vi "Test.vi"() -> ()   [LabVIEW 2014]
panel:
  out "PLC连线成功":bool
  out "接收数据":string
  # "8000 0200 0100 00C0 0000 0101 8207 D000 0001"
  # "C0 00 02 00 C0 00 00 01 00 00 01 01 00 00 00 54"
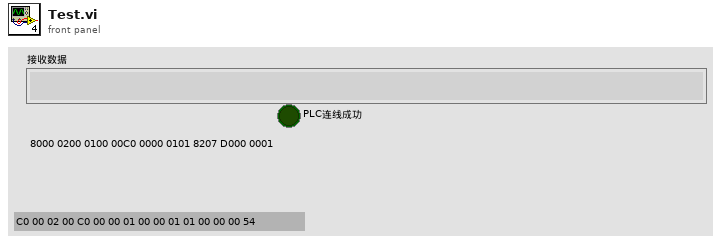
[diagram p1: front panel]
types:
  T1 = typedef "欧姆龙PLC Action.ctl" = enum16{"初始化", "重新初始化", "读触发信息", "读示教坐标信息", "写数据", "获取信息"}
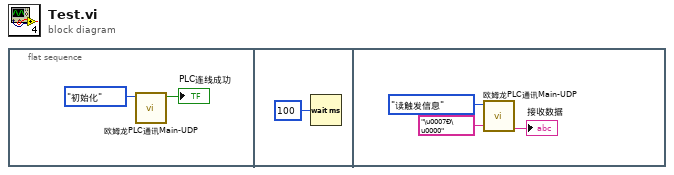
[diagram p0: block diagram]
diagram:
  n1 = flat-sequence {
    frame #0 {
      n2 = call "欧姆龙PLC通讯Main-UDP.vi"("欧姆龙PLC Action"=欧姆龙PLC_Action."初始化") -> ("PLC连线成功"=→"PLC连线成功":bool)  [unwired: 8 in, 2 out]
    }
    frame #1 {
      n3 = Wait (ms)(milliseconds to wait=u32 100 ("等待时间（毫秒）")) -> ()  [unwired: 1 out]
    }
    frame #2 {
      n4 = call "欧姆龙PLC通讯Main-UDP.vi"("起始地址"="\u0007Ð\u0000", "欧姆龙PLC Action"=欧姆龙PLC_Action."读触发信息") -> ("接收数据"=→"接收数据":string)  [unwired: 7 in, 2 out]
    }
  }
